vi "VerifyJUnitReportPath.vi"(8 "error in (no error)":errorcluster, 11 "RunUnitTests in":refnum<class "RunUnitTests.lvclass">) -> (0 "error out":errorcluster, 3 "RunUnitTests out":refnum<class "RunUnitTests.lvclass">)   [LabVIEW 2014, in "RunUnitTests.lvclass"]
uses:
  RunUnitTests.lvclass
  RunUnitTests.lvclass/RunUnitTests.ctl
  Utilities/OperationErrorType.ctl
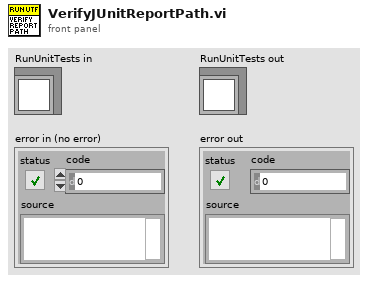
[diagram p1: front panel]
types:
  T1 = typedef "OperationErrorType.ctl" = enum16{"RequiredArgumentMissing", "UnknownArguments", "LoggerSetMultipleTimes", "OperationBrokenError"}
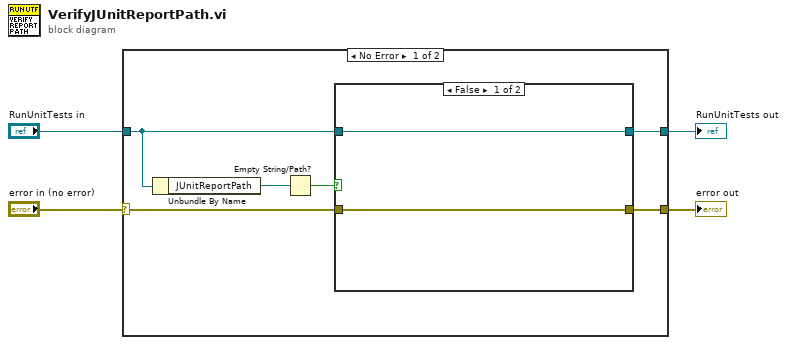
[diagram p0: block diagram]
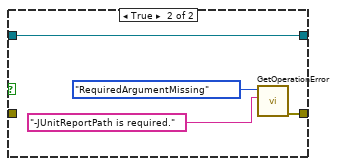
[diagram p2: hidden frame]
diagram:
  n1 = case shown="No Error" "error in (no error)" {
    selector: "error in (no error)" -> [w10 w17]
    tunnel: [w9 w18] -> w2
    tunnel: "RunUnitTests in" -> [w8 w18]
    tunnel: [w7 w17] -> w4
    frame No Error {
      n2 = Unbundle By Name(w8) -> ("JUnitReportPath"=w6:path)
      n3 = Empty String/Path?(string/path=w6) -> (empty?=w5:bool)
      n4 = case shown="False" w5 {
        tunnel: w10 -> [w11 _]
        tunnel: [w12 w16] -> w9
        tunnel: w8 -> [w12 w16]
        tunnel: [w11 w13] -> w7
        frame False {
        }
        frame True {
          n5 = call "GetOperationError.vi"("Additional Information"="-JUnitReportPath is required.", "Operation Error Type"=OperationErrorType."RequiredArgumentMissing") -> ("error out"=w13:errorcluster)  [unwired: 9 in]
        }
      }
    }
    frame Error {
    }
  }
  "error out" <- w4
  "RunUnitTests out" <- w2
